vi "source.get.vi"(8 "error in (no error)":errorcluster, 11 "datasource in":refnum<class "datasource.lvclass">) -> (0 "error out":errorcluster, 2 "datasources.lvlib:source.lvclass":refnum<class "source.lvclass">, 3 "datasource out":refnum<class "datasource.lvclass">)   [LabVIEW 2020, in "datasources.lvlib" / "datasource.lvclass"]
uses:
  datasource.lvclass
  source/source.lvclass
  datasource.lvclass/datasource.ctl
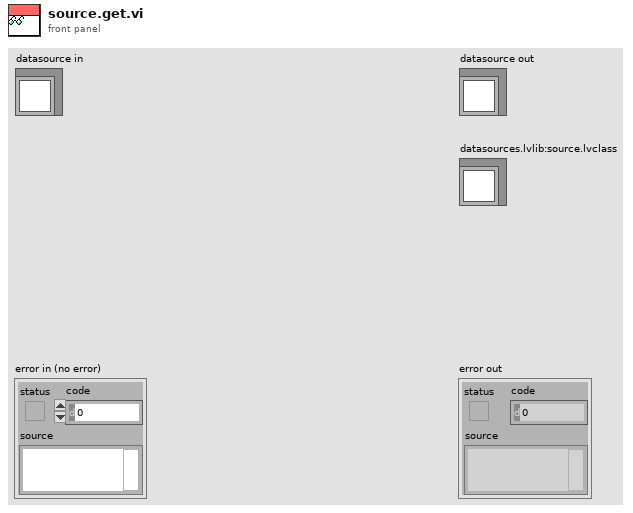
[diagram p1: front panel]
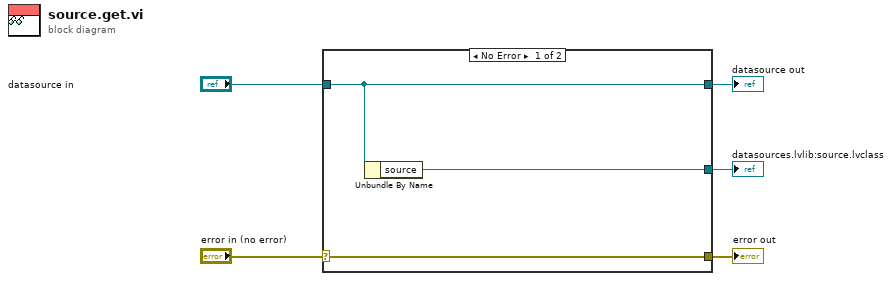
[diagram p0: block diagram]
diagram:
  n1 = case shown="No Error" "error in (no error)" {
    selector: "error in (no error)" -> [w8 w9]
    tunnel: [w8 w9] -> w4
    tunnel: [w7 w10] -> w2
    tunnel: "datasource in" -> [w7 w10]
    tunnel: [w6 _] -> w1
    frame No Error {
      n2 = Unbundle By Name(w7) -> ("source"=w6:refnum<class "source.lvclass">)
    }
    frame Error {
    }
  }
  "error out" <- w4
  "datasource out" <- w2
  "datasources.lvlib:source.lvclass" <- w1
